vi "tcsWEP_getEvent_normalTargetWfsList.vi"(8 "error in (no error)":errorcluster, 11 "logevent_normalTargetWfsList_Ctl":T1={"sensorIdList[4]"=[0, 0, 0, 0], "timestamp"=0.0, "priority"=0}) -> (0 "error out":errorcluster, 2 "function return":i32, 3 "logevent_normalTargetWfsList_Ctl out":T1)   [LabVIEW 2016, in "SALLV_tcsWEP.lvlib"]
doc: "int tcsWEP_shm_getEvent_normalTargetWfsListLV(tcsWEP_logevent_normalTargetWfsListLV *logevent_normalTargetWfsList_Ctl );"
uses:
  SALLV_tcsWEP.lvlib
  DataTypes/logevent_normalTargetWfsList.ctl
  SALLV_tcsWEP.so
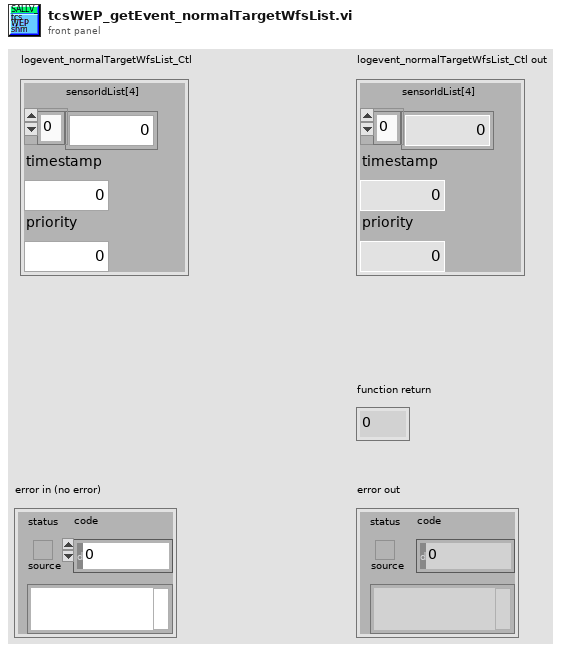
[diagram p1: front panel]
types:
  T1 = typedef "SALLV_tcsWEP.lvlib/logevent_normalTargetWfsList.ctl" = cluster{"sensorIdList[4]":i16[], "timestamp":dbl, "priority":i32}
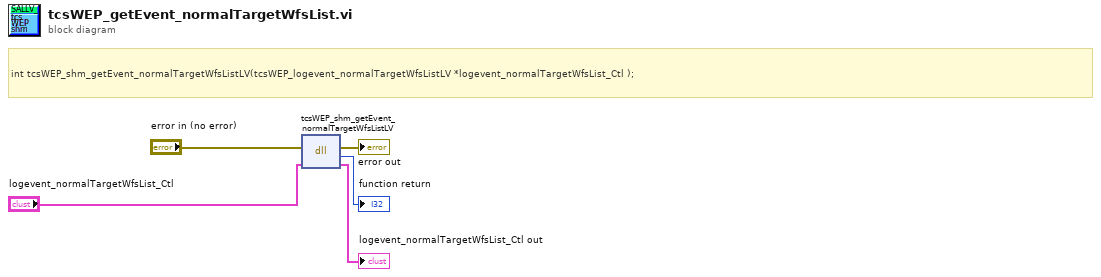
[diagram p0: block diagram]
diagram:
  # "int tcsWEP_shm_getEvent_normalTargetWfsListLV(tcsWEP_logevent_normalTargetWfsListLV *logevent_normalTargetWfsList_Ctl );"
  n1 = dll-call lib="home/ttsai/Documents/salAPI/SALLV_tcsWEP.*" fn="tcsWEP_shm_getEvent_normalTargetWfsListLV"(error in="error in (no error)", "logevent_normalTargetWfsList_Ctl"="logevent_normalTargetWfsList_Ctl") -> (error out=→"error out":errorcluster, →"function return":i32, "logevent_normalTargetWfsList_Ctl"=→"logevent_normalTargetWfsList_Ctl out":T1)  [unwired: 2 in, 1 out]
